vi "Free Pixels with Chances.vi"(10 "indices":T1, 11 "Picture in":refnum<class "Picture.lvclass">) -> (0 "Empty?":bool, 2 "Free Pixels":cluster{"Weight":dbl, "indices":T1}[](array[cluster]), 3 "Picture out":refnum<class "Picture.lvclass">)   [LabVIEW 2018]
uses:
  Picture.lvclass
  Coords.ctl
  Picture.lvclass/Picture.ctl
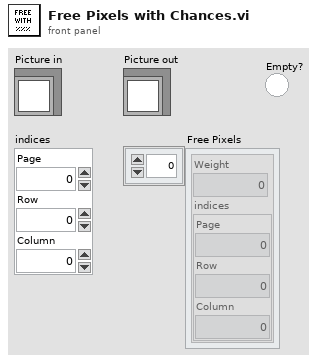
[diagram p1: front panel]
types:
  T1 = typedef "Coords.ctl" = cluster{"Page":i32, "Row":i32, "Column":i32}
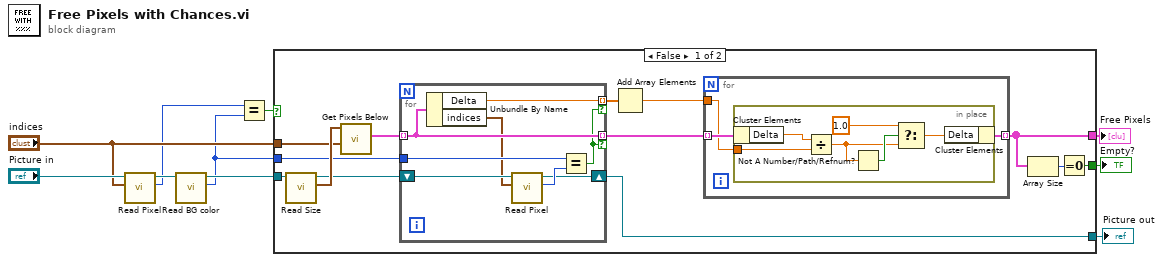
[diagram p0: block diagram]
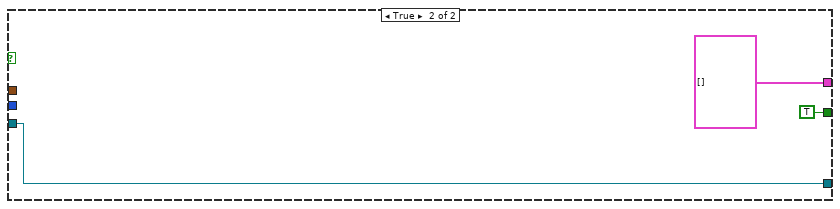
[diagram p2: hidden frame]
diagram:
  n1 = call "Read Pixel.vi"("indices"="indices", "Picture in"="Picture in") -> ("Color"=w3:u32, "Picture out"=w5:refnum<class "Picture.lvclass">)  [unwired: 7 in, 1 out]
  n2 = call "Read BG color.vi"("Picture in"=w5) -> ("BG color"=w2:u32, "Picture out"=w4:refnum<class "Picture.lvclass">)  [unwired: 8 in, 1 out]
  n3 = Equal?(x=w3, y=w2) -> (x = y?=w1:bool)
  n4 = case shown="False" w1 {
    tunnel: [w23 w43] -> w10
    tunnel: [w18 cluster{"Delta":dbl, "indices":T1}[] []] -> w9
    tunnel: [w16 TRUE] -> w8
    tunnel: "indices" -> [w14 _]
    tunnel: w4 -> [w13 w43]
    tunnel: w2 -> [w11 _]
    frame False {
      n5 = call "Read Size.vi"("Picture in"=w13) -> ("Pixmap Size"=w19:T1, "Picture out"=w12:refnum<class "Picture.lvclass">)  [unwired: 8 in, 1 out]
      n6 = call "Get Pixels Below.vi"("Pixel"=w14, "Pixmap Size"=w19) -> ("Pixels Below"=w20:cluster{"Delta":dbl, "indices":T1}[])  [unwired: 9 in]
      n7 = for {
        tunnel: w20 -> [w39] mode=indexing
        tunnel: w11 -> [w37]
        tunnel: [w39] -> w15 mode=indexing if=w34
        tunnel: [w35] -> w21 mode=indexing if=w34
        shift-right: [w33] -> w23
        shift-left: w12 -> [w40]
        n8 = Unbundle By Name(w39) -> ("Delta"=w35:dbl, "indices"=w36:T1)
        n9 = call "Read Pixel.vi"("indices"=w36, "Picture in"=w40) -> ("Color"=w38:u32, "Picture out"=w33:refnum<class "Picture.lvclass">)  [unwired: 7 in, 1 out]
        n10 = Equal?(x=w37, y=w38) -> (x = y?=w34:bool)
      }
      n11 = Add Array Elements(numeric array=w21) -> (sum=w22:dbl)
      n12 = for {
        tunnel: w15 -> [w26] mode=indexing
        tunnel: w22 -> [w25]
        tunnel: [w24] -> w18 mode=indexing
        n13 = in-place {
          in-place-border: w25 -> [w27]
          n14 = in-place-cluster #1(w26) -> ("Delta"=w29:dbl)
          n15 = Divide(x=w29, y=w27) -> (x/y=w30:dbl)
          n16 = Not A Number/Path/Refnum?(number/path/refnum=w30) -> (NaN/Path/Refnum?=w32:bool)
          n17 = Select(t=1.0, s=w32, f=w30) -> (s? t:f=w28:dbl)
          n18 = in-place-cluster #1("Delta"=w28) -> (w24:cluster{"Delta":dbl, "indices":T1})
        }
      }
      n19 = Array Size(array=w18) -> (size(s)=w17:i32)
      n20 = Equal To 0?(x=w17) -> (x = 0?=w16:bool)
    }
    frame True {
    }
  }
  "Picture out" <- w10
  "Free Pixels" <- w9
  "Empty?" <- w8
